vi "writeMasterBatch.vi"(4 "ROI Parameters":T1, 6 "Drop Time (ms)":dbl, 7 "file (use dialog)":path, 8 "Master Batch 5th":dbl, 9 "Master Batch 4th":dbl, 10 "Master Batch 3rd":dbl, 11 "Scan name":string) -> ()   [LabVIEW 2016]
uses:
  Controls/ScanParameters/ROI_set.ctl
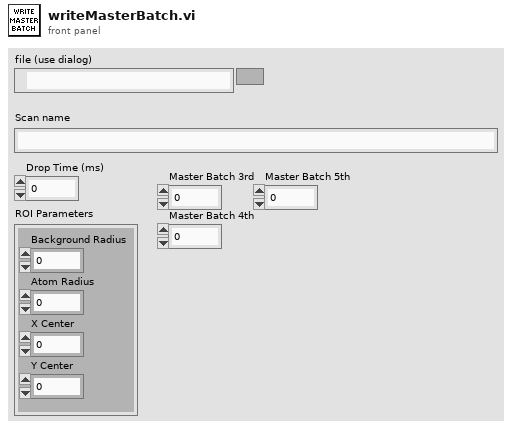
[diagram p1: front panel]
types:
  T1 = typedef "ROI_set.ctl" = cluster{"Background Radius":dbl, "Atom Radius":dbl, "X Center":dbl, "Y Center":dbl}
  T2 = enum16{"open", "replace", "create", "open or create", "replace or create", "replace or create with confirmation"}
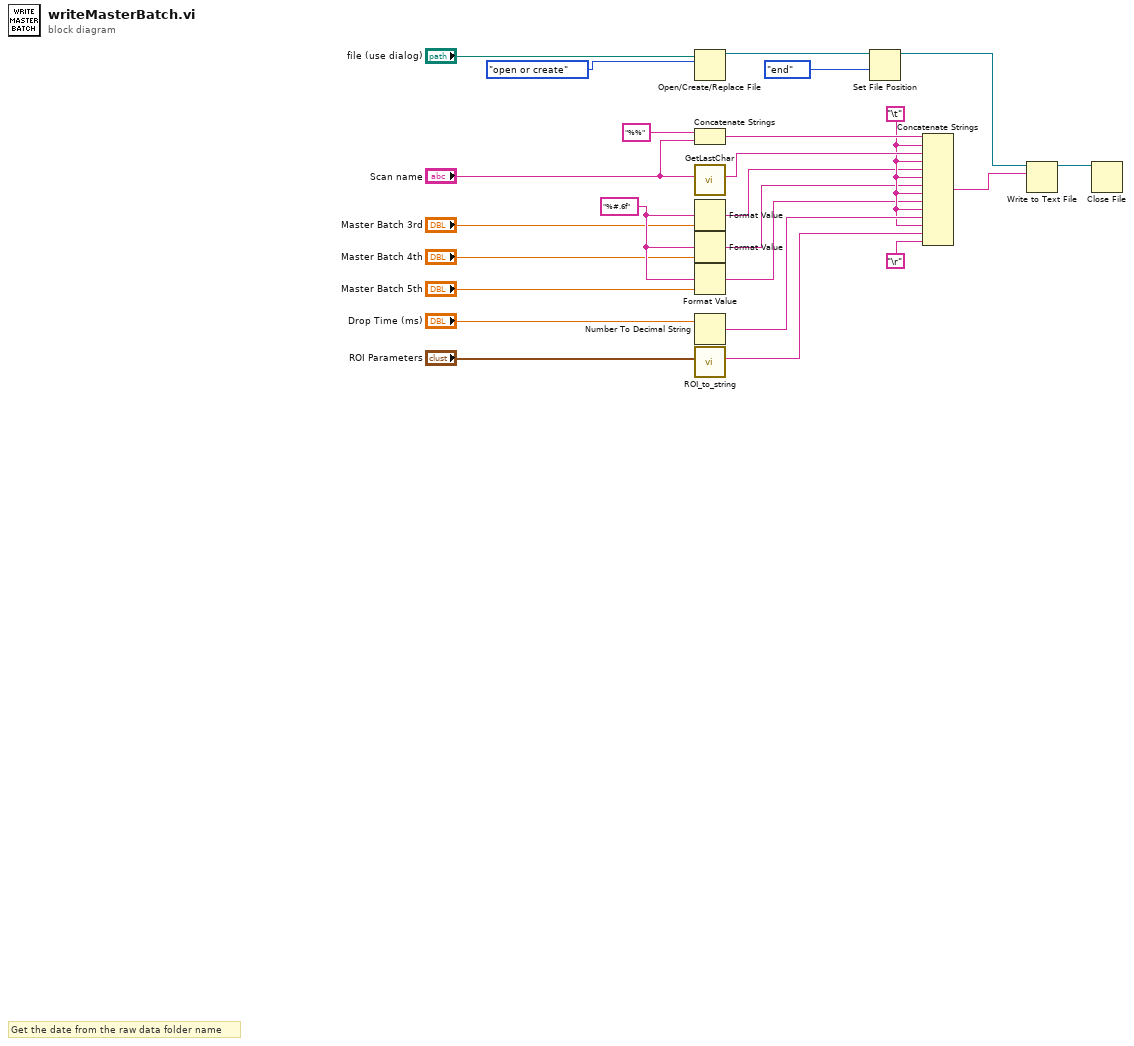
[diagram p0: block diagram]
diagram:
  w4 = "%#.6f" ("format string")
  w9 = "\t"
  # "Get the date from the raw data folder name"
  n1 = Open/Create/Replace File(file path (use dialog)="file (use dialog)", operation (0:open)=T2."open or create") -> (refnum out=w13:refnum<file>)  [unwired: 4 in, 2 out]
  n2 = Concatenate Strings("%%" ("string"), "Scan name") -> (w16:string)
  n3 = call "GetLastChar.vi"("String"="Scan name") -> ("String 2"=w21:string)  [unwired: 10 in]
  n4 = Format Value(format string=w4, value (0)="Master Batch 3rd") -> (output string=w8:string)  [unwired: 1 in]
  n5 = Format Value(format string=w4, value (0)="Master Batch 4th") -> (output string=w7:string)  [unwired: 1 in]
  n6 = Format Value(format string=w4, value (0)="Master Batch 5th") -> (output string=w6:string)  [unwired: 1 in]
  n7 = Number To Decimal String(number="Drop Time (ms)") -> (decimal integer string=w19:string)  [unwired: 1 in]
  n8 = call "ROI_to_string.vi"("ROI Parameters"="ROI Parameters") -> ("String"=w20:string)  [unwired: 10 in]
  n9 = Set File Position(refnum=w13, from (0:start)=enum16{"start", "end", "current"}."end") -> (refnum out=w11:refnum<file>)  [unwired: 2 in, 1 out]
  n10 = Concatenate Strings(w16, w9, w21, w9, w8, w9, w7, w9, w6, w9, w19, w9, w20, "\r") -> (w22:string)
  n11 = Write to Text File(file (use dialog)=w11, text=w22) -> (refnum out=w10:refnum<file>)  [unwired: 2 in, 2 out]
  n12 = Close File(refnum=w10) -> ()  [unwired: 1 in, 2 out]
